vi "Find Compatible Hardware for Measurement.vi"(8 "error in (no error)":errorcluster, 10 "Measurement Name":string, 11 "Controller in":refnum<class "Controller.lvclass">) -> (0 "error out":errorcluster, 3 "Controller out":refnum<class "Controller.lvclass">)   [LabVIEW 2016, in "Controller Actor.lvlib" / "Controller.lvclass"]
uses:
  Controller.lvclass
  C:/Program Files (x86)/National Instruments/LabVIEW 2016/vi.lib/ActorFramework/Actor/Actor.lvclass
  <vilib>/ActorFramework/Actor/Actor.lvclass/Actor.ctl
  <vilib>/ActorFramework/Message Enqueuer/Message Enqueuer.lvclass/Message Enqueuer.ctl
  Messages/Find Devices of Specified Type Msg/Find Devices of Specified Type Msg.lvclass/Find Devices of Specified Type Msg.ctl
  <vilib>/ActorFramework/Message Enqueuer/Init from Existing Queue.vi
  <vilib>/ActorFramework/Message Enqueuer/Enqueue.vi
  Messages/Find Devices of Specified Type Msg/Find Devices of Specified Type Msg.lvclass
  C:/Program Files (x86)/National Instruments/LabVIEW 2016/vi.lib/ActorFramework/Message/Message.lvclass
  <vilib>/ActorFramework/Message Priority Queue/Priority Enqueue.vi
  <vilib>/ActorFramework/Message Enqueuer/Message Enqueuer.lvclass
  Measurement Actor/Measurement.lvclass
  <vilib>/ActorFramework/Actor/Actor.lvclass
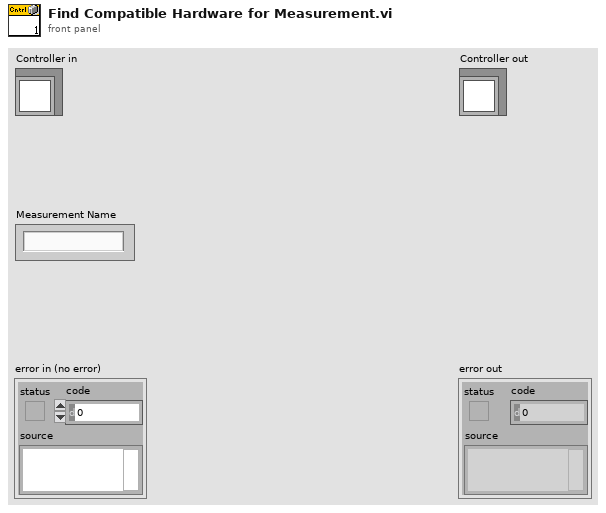
[diagram p1: front panel]
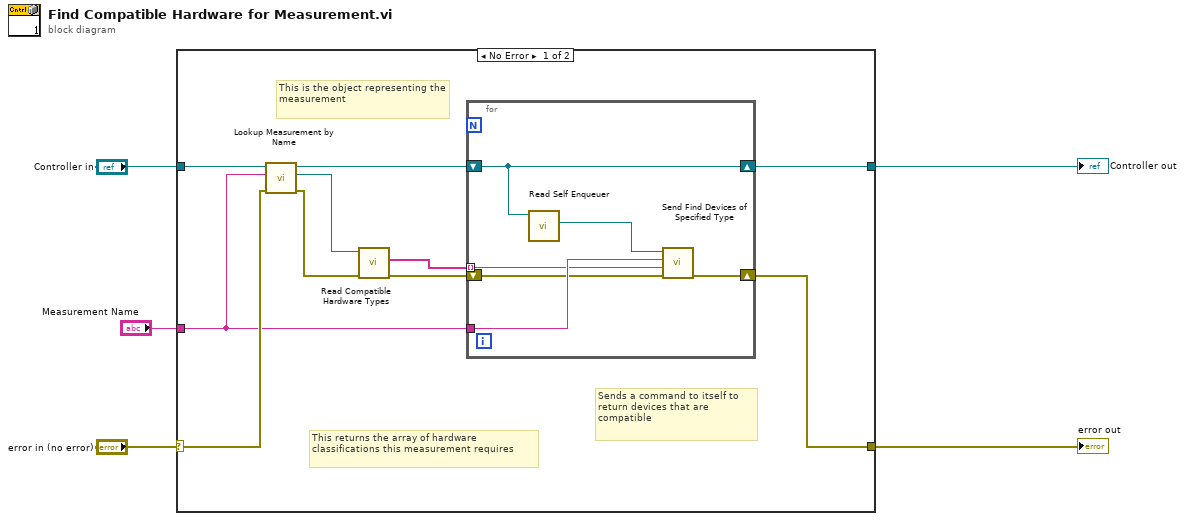
[diagram p0: block diagram]
diagram:
  n1 = case shown="No Error" "error in (no error)" {
    selector: "error in (no error)" -> [w8 w22]
    tunnel: [w7 w22] -> w4
    tunnel: [w11 w21] -> w1
    tunnel: "Controller in" -> [w15 w21]
    tunnel: "Measurement Name" -> [w6 _]
    frame No Error {
      # "Sends a command to itself to return devices that are compatible"
      # "This returns the array of hardware classifications this measurement requires"
      # "This is the object representing the measurement"
      n2 = call "Lookup Measurement by Name.vi"("error in (no error)"=w8, "Measurement Name"=w6, "Controller in"=w15) -> ("error out"=w9:errorcluster, "Measurement.lvclass"=w14:refnum<class "Measurement.lvclass">, "Controller out"=w13:refnum<class "Controller.lvclass">)  [unwired: 5 in, 1 out]
      n3 = call-dynamic "Read Compatible Hardware Types.vi"("error in (no error)"=w9, "Measurement in"=w14) -> ("error out"=w10:errorcluster, "Compatible Hardware Types"=w12:string[])  [unwired: 7 in, 1 out]
      n4 = for {
        tunnel: w12 -> [w19] mode=indexing
        shift-right: [w18] -> w11
        shift-left: w13 -> [w18]
        shift-right: [w16] -> w7
        shift-left: w10 -> [w16]
        tunnel: w6 -> [w20]
        n5 = call <vilib>:"Read Self Enqueuer.vi"("Actor"=w18) -> ("Self Enqueuer"=w17:refnum<class "Message Enqueuer.lvclass">)  [unwired: 10 in]
        n6 = call "Send Find Devices of Specified Type.vi"("error in (no error)"=w16, "Hardware Type"=w19, "Measurement Name"=w20, "Message Enqueuer"=w17) -> ()  [unwired: 6 in, 2 out]
      }
    }
    frame Error {
    }
  }
  "error out" <- w4
  "Controller out" <- w1
